vi "CalculateAmplitudeModulation_1.vi"(5 "b_am":fxp<+/-,16,2>, 7 "a_am":fxp<+/-,16,2>, 8 "input valid":bool=TRUE, 9 "cos_am":fxp<+/-,16,0>, 11 "Data in":fxp<+/-,16,14>[](array[numeric])=[0.0, 0.0]) -> (0 "output valid":bool, 3 "Data out":fxp<+/-,16,14>[](array[numeric]))   [LabVIEW 2013]
doc: "Calculates various combinations on I_in, Q_in and cos(fi) and sin(fi) to be used later to delay the output signal"
uses:
  <vilib>/rvi/FXPMathLib/FxpInterpret/XNode/nifxpmath_Interpret.xnode
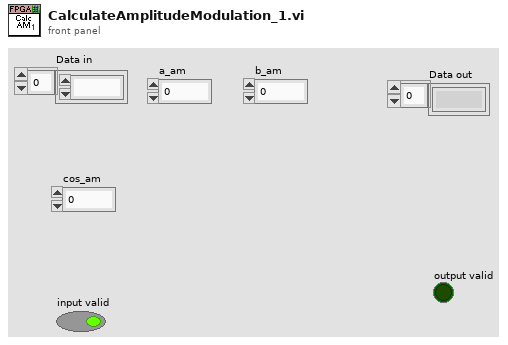
[diagram p1: front panel]
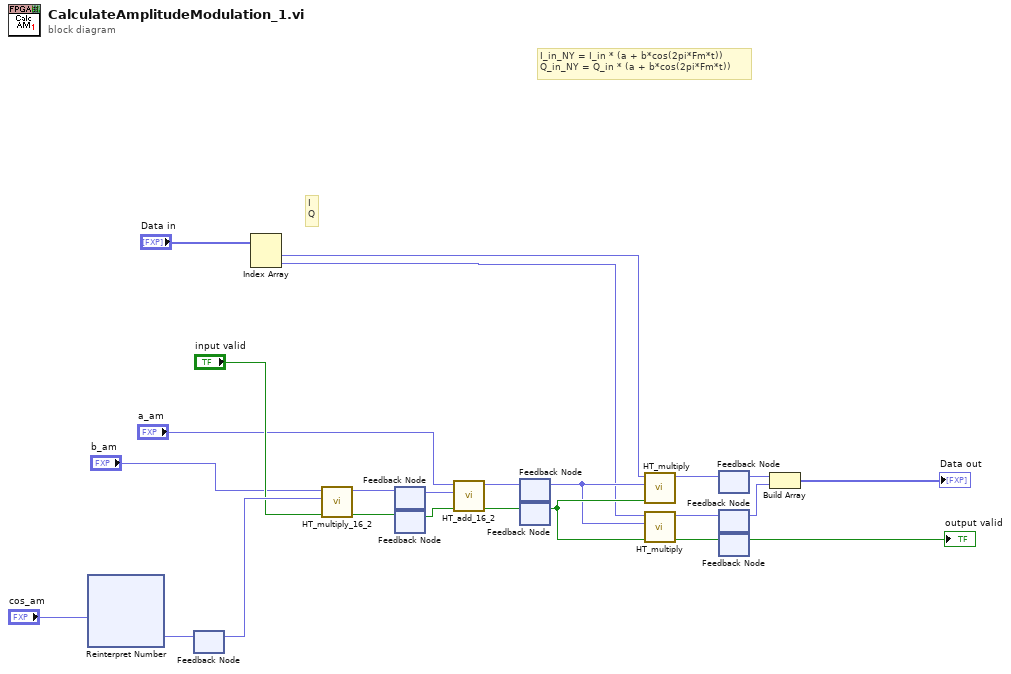
[diagram p0: block diagram]
diagram:
  # "I\nQ"
  # "I_in_NY = I_in * (a + b*cos(2pi*Fm*t))\nQ_in_NY = Q_in * (a + b*cos(2pi*Fm*t))"
  n1 = xnode "Reinterpret Number"("x"="cos_am") -> ("y"=w22:fxp<+/-,16,2>)
  n2 = feedback #1() -> (w21:fxp<+/-,16,2>)  [unwired: 1 in]
  n3 = feedback-in #1(w22) -> ()
  n4 = Index Array(array="Data in") -> (element #1=w9:fxp<+/-,16,14>, element #2=w8:fxp<+/-,16,14>)  [unwired: 2 in]
  n5 = call "HT_multiply_16_2.vi"("input valid"="input valid", "y"=w21, "x"="b_am") -> ("output valid"=w16:bool, "x*y"=w17:fxp<+/-,16,2>)  [unwired: 7 in]
  n6 = feedback #2() -> (w15:fxp<+/-,16,2>)  [unwired: 1 in]
  n7 = feedback-in #2(w17) -> ()
  n8 = feedback #3() -> (w14:bool)  [unwired: 1 in]
  n9 = feedback-in #3(w16) -> ()
  n10 = call "HT_add_16_2.vi"("input valid"=w14, "y"=w15, "x"="a_am") -> ("output valid"=w13:bool, "x+y"=w12:fxp<+/-,16,2>)  [unwired: 7 in]
  n11 = feedback #4() -> (w10:fxp<+/-,16,2>)  [unwired: 1 in]
  n12 = feedback-in #4(w12) -> ()
  n13 = feedback #5() -> (w11:bool)  [unwired: 1 in]
  n14 = feedback-in #5(w13) -> ()
  n15 = call "HT_multiply.vi"("input valid"=w11, "y"=w10, "x"=w9) -> ("x*y"=w7:fxp<+/-,16,14>)  [unwired: 7 in, 1 out]
  n16 = call "HT_multiply.vi"("input valid"=w11, "y"=w10, "x"=w8) -> ("output valid"=w1:bool, "x*y"=w6:fxp<+/-,16,14>)  [unwired: 7 in]
  n17 = feedback #6() -> (w4:fxp<+/-,16,14>)  [unwired: 1 in]
  n18 = feedback-in #6(w7) -> ()
  n19 = feedback #7() -> (w3:fxp<+/-,16,14>)  [unwired: 1 in]
  n20 = feedback-in #7(w6) -> ()
  n21 = feedback #8() -> (→"output valid":bool)  [unwired: 1 in]
  n22 = feedback-in #8(w1) -> ()
  n23 = Build Array(w4, w3) -> (→"Data out":fxp<+/-,16,14>[])
